vi "ChargePump_Core.vi"(8 "error in (no error)":errorcluster, 10 "Core PLL Instance":string(combo)="Core0", 11 "Charge Pump Setting":string(combo)="Normal") -> (0 "error out":errorcluster)   [LabVIEW 2011]
doc: "This VI sets the charge pump to the desired state for the instance of the Core PLL selected.\n\nInputs:\n1. Charge Pump Setting: Sets the charge pump to the desire state (Normal or Down).\n2. Core PLL Instance: Instance of the Core PLL to to have Charge Pump set (Core0, Core1, etc.)."
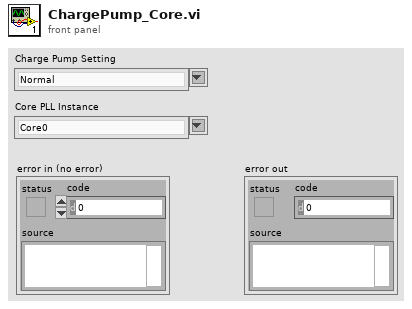
[diagram p1: front panel]
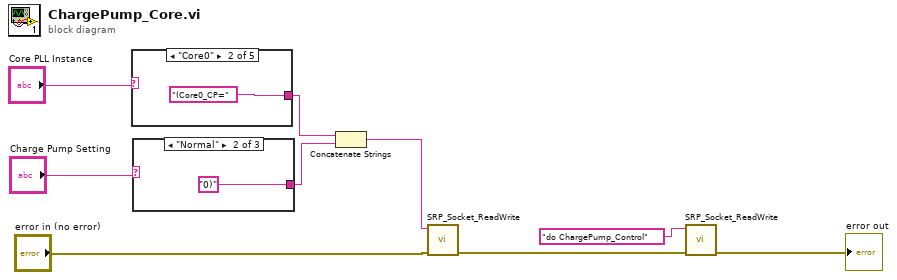
[diagram p0: block diagram]
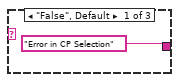
[diagram p2: hidden frame]
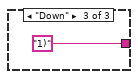
[diagram p3: hidden frame]
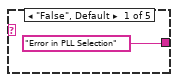
[diagram p4: hidden frame]
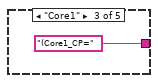
[diagram p5: hidden frame]
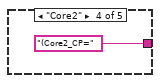
[diagram p6: hidden frame]
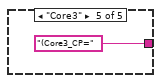
[diagram p7: hidden frame]
diagram:
  n1 = case shown="\"Core0\"" "Core PLL Instance" {
    tunnel: ["Error in PLL Selection" "(Core0_CP=" "(Core1_CP=" "(Core2_CP=" "(Core3_CP="] -> w7
    frame "False", Default {
    }
    frame "Core0" {
    }
    frame "Core1" {
    }
    frame "Core2" {
    }
    frame "Core3" {
    }
  }
  n2 = case shown="\"Normal\"" "Charge Pump Setting" {
    tunnel: ["Error in CP Selection" "0)" "1)"] -> w6
    frame "False", Default {
    }
    frame "Normal" {
    }
    frame "Down" {
    }
  }
  n3 = Concatenate Strings(w7, w6) -> (w4:string)
  n4 = call "SRP_Socket_ReadWrite.vi"("error in (no error)"="error in (no error)", "Data In"=w4) -> ("error out"=w5:errorcluster)  [unwired: 7 in, 1 out]
  n5 = call "SRP_Socket_ReadWrite.vi"("error in (no error)"=w5, "Data In"="do ChargePump_Control") -> ("error out"=→"error out":errorcluster)  [unwired: 7 in, 1 out]
